vi "Filter_on_template_file_new.vi"(0 "Template File":path, 2 "Extra Channel Values":string[][](array[string]), 3 "Filetype":string, 5 "Channel Names In":string[](array[string]), 9 "Data string":string, 12 "Filename":path) -> (4 "Template File-write":path, 6 "Row numbers":i32[](array[numeric]), 10 "Channel Names Out":string[](array[string]), 14 "Deleted Rows":string[][](array[string]), 15 "Data Out":string[][](array[string]))   [LabVIEW 2021]
panel:
  out "Current Case":string
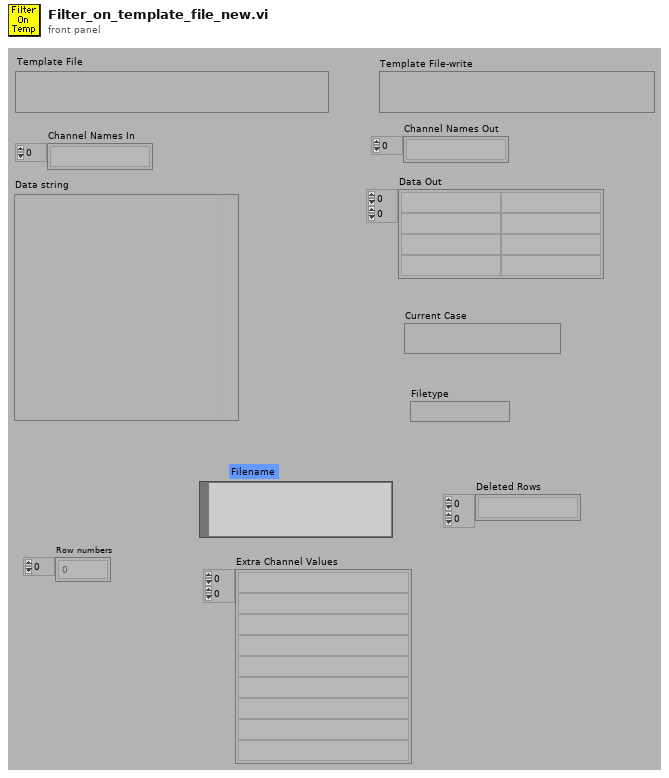
[diagram p1: front panel]
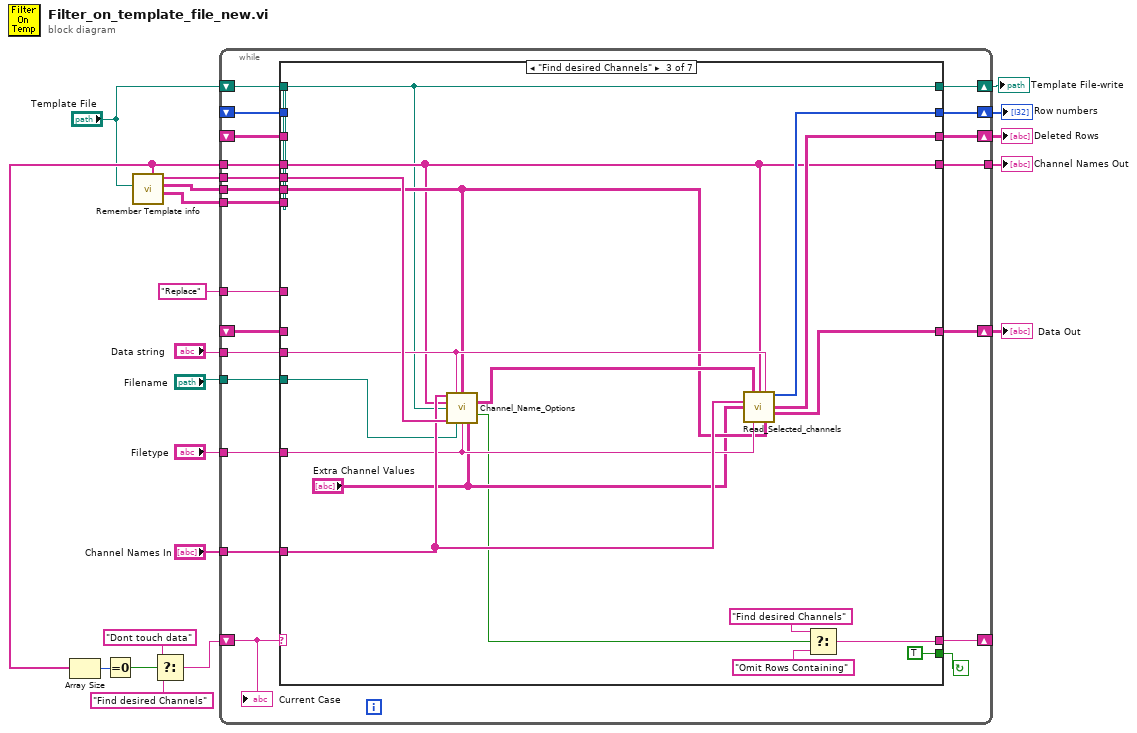
[diagram p0: block diagram]
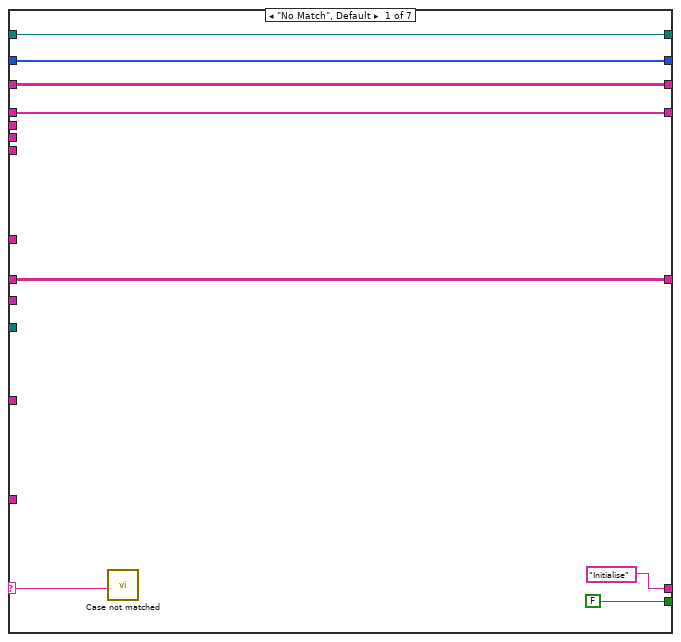
[diagram p2: hidden frame]
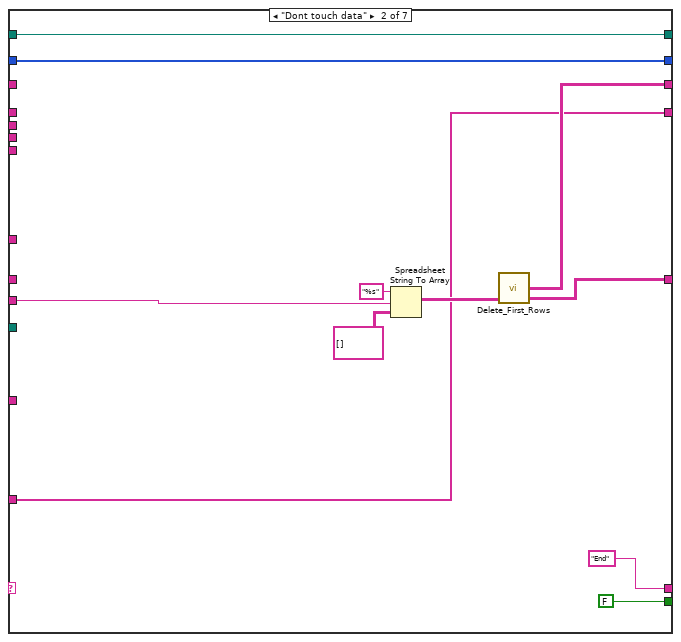
[diagram p3: hidden frame]
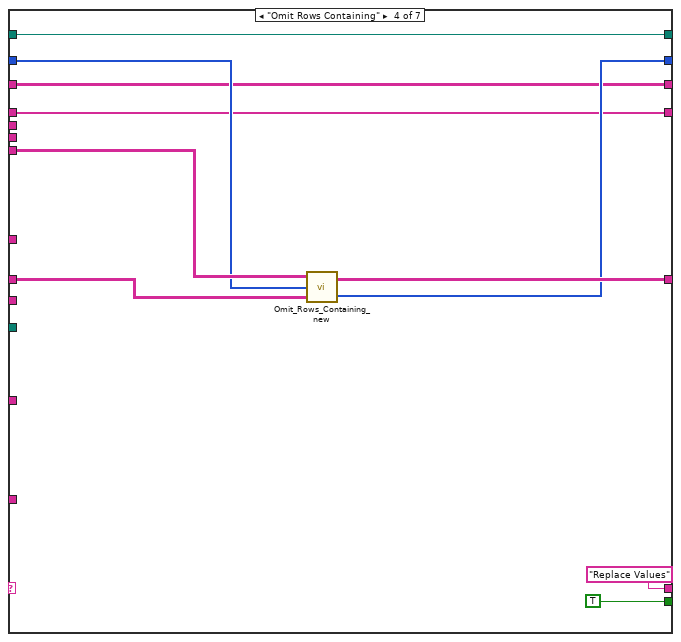
[diagram p4: hidden frame]
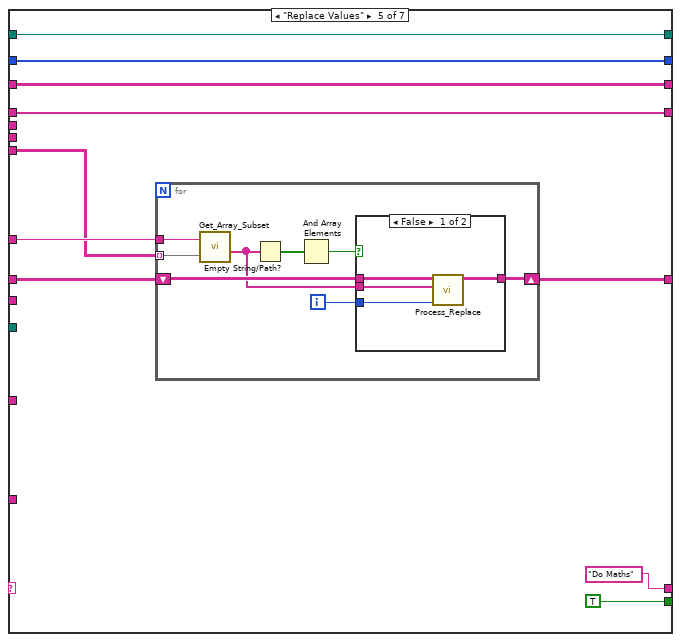
[diagram p5: hidden frame]
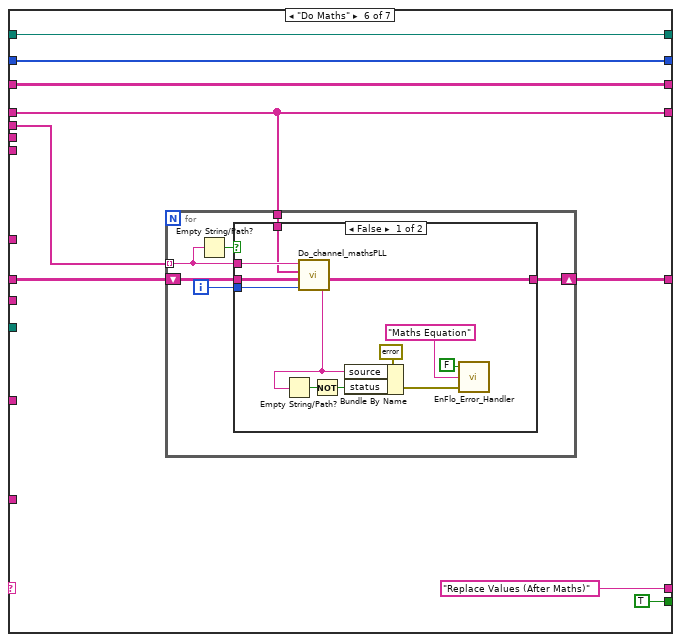
[diagram p7: hidden frame]
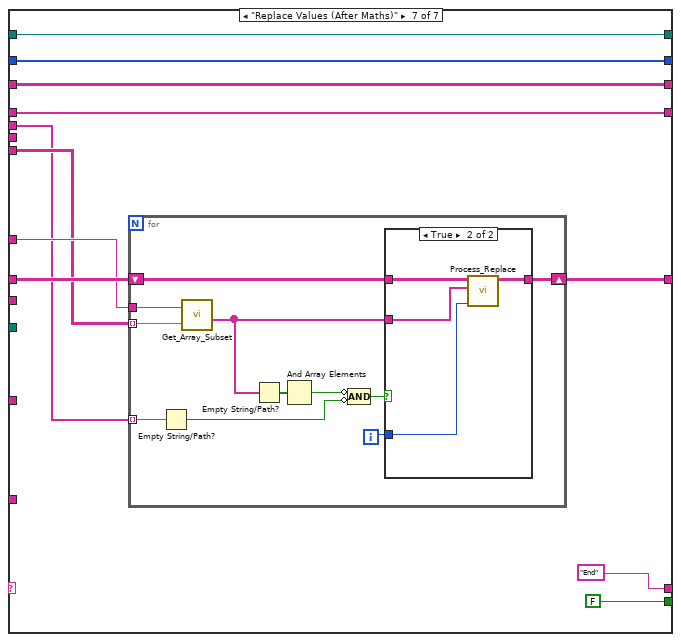
[diagram p9: hidden frame]
diagram:
  n1 = call "Remember Template info.vi"("Template File"="Template File") -> ("2D Template info"=w9:string[][], "Ignore"=w11:string[][], "Maths"=w10:string[], "Template Ch Names Out"=w8:string[])  [unwired: 6 in, 1 out]
  n2 = Array Size(array=w8) -> (size(s)=w7:i32)
  n3 = Equal To 0?(x=w7) -> (x = 0?=w6:bool)
  n4 = Select(t="Dont touch data", s=w6, f="Find desired Channels") -> (s? t:f=w4:string)
  n5 = while {
    tunnel: "Filetype" -> [w21]
    tunnel: "Filename" -> [w32]
    tunnel: "Data string" -> [w33]
    tunnel: "Channel Names In" -> [w34]
    tunnel: "Replace" -> [w35]
    shift-left: _ -> [w36]
    shift-right: [w37] -> w18
    shift-left: "Template File" -> [w38]
    shift-right: [w39] -> w20
    shift-left: w4 -> [w31]
    shift-right: [w40] -> _
    shift-right: [w29] -> w13
    shift-left: _ -> [w30]
    shift-right: [w28] -> w12
    shift-left: _ -> [w27]
    tunnel: w11 -> [w26]
    tunnel: w10 -> [w25]
    tunnel: w9 -> [w24]
    tunnel: w8 -> [w23]
    tunnel: [w22] -> w2
    stop <- w41 continue-if-true
    n6 = case shown="\"Find desired Channels\"" w31 {
      selector: w31 -> [w43 _ _ _ _ _ _]
      tunnel: [FALSE FALSE ("Duplicate rows?") TRUE TRUE TRUE TRUE ("Duplicate rows?") FALSE] -> w41
      tunnel: ["Initialise" "End" w63 "Replace Values" "Do Maths" "Replace Values (After Maths)" "End"] -> w40
      tunnel: [w47 w60 w62 w86 w96 w120 w148] -> w39
      tunnel: w24 -> [_ _ _ w85 w91 _ w143]
      tunnel: w38 -> [w47 w60 w62 w86 w96 w120 w148]
      tunnel: w25 -> [_ _ w77 _ _ w119 w142]
      tunnel: [w46 w53 w74 w83 w95 w115 w147] -> w37
      tunnel: w36 -> [w46 _ _ w84 w94 w116 w146]
      tunnel: w35 -> [_ _ _ _ w92 _ w144]
      tunnel: w34 -> [_ w50 w76 _ _ _ _]
      tunnel: w33 -> [_ w55 w72 _ _ _ _]
      tunnel: w32 -> [_ _ w61 _ _ _ _]
      tunnel: w21 -> [_ _ w73 _ _ _ _]
      tunnel: [w45 w52 w71 w82 w93 w114 w145] -> w29
      tunnel: w30 -> [w45 w52 _ w81 w93 w114 w145]
      tunnel: [w44 w51 w70 w80 w90 w113 w141] -> w28
      tunnel: w27 -> [w44 _ _ w80 w90 w113 w141]
      tunnel: w26 -> [_ _ w69 _ _ _ _]
      tunnel: w23 -> [w42 _ w68 w79 w89 w112 w140]
      tunnel: [w42 w50 w68 w79 w89 w112 w140] -> w22
      frame "No Match", Default {
        n7 = call "Case not matched.vi"("Case Name not Matched"=w43) -> ()
      }
      frame "Dont touch data" {
        n8 = Spreadsheet String To Array(format string="%s", spreadsheet string=w55, array type (2D Dbl)=string[][] [] ("Channel Values")) -> (array=w54:string[][])  [unwired: 1 out]
        n9 = call "Delete_First_Rows.vi"("Data In"=w54) -> ("Deleted Rows"=w51:string[][], "Data Out"=w53:string[][])  [unwired: 1 in, 1 out]
      }
      frame "Find desired Channels" {
        n10 = call "Channel_Name_Options.vi"("All Channel Names"=w76, "Data string"=w72, "Ignore When"=w69, "Template Names"=w68, "Template File"=w62, "Maths In"=w77, "while Reading:"=w61, "Filetype"=w73, "Extra Channel Values"="Extra Channel Values") -> ("Valid Channel Options"=w75:string[][], "Template updated?"=w66:bool)  [unwired: 5 out]
        n11 = call "Read_Selected_channels.vi"("Valid Channel Options"=w75, "Template Names"=w68, "Data string"=w72, "All Channels Present"=w76, "Extra Channels"="Extra Channel Values", "Filetype"=w73, "Ignore When"=w69) -> ("Non-Blank Rows"=w71:i32[], "Deleted Rows"=w70:string[][], "Output Values"=w74:string[][])  [unwired: 5 in, 1 out]
        n12 = Select(t="Find desired Channels", s=w66, f="Omit Rows Containing") -> (s? t:f=w63:string)
      }
      frame "Omit Rows Containing" {
        n13 = call "Omit_Rows_Containing_new.vi"("Data Array In"=w84, "Non-Blank Rows"=w81, "Template Info"=w85) -> ("Row numbers"=w82:i32[], "Data Array Out"=w83:string[][])
      }
      frame "Replace Values" {
        n14 = for {
          shift-right: [w104] -> w95
          shift-left: w94 -> [w105]
          tunnel: w92 -> [w101]
          tunnel: w91 -> [w100] mode=indexing
          i -> [w106]
          n15 = call "Get_Array_Subset.vi"("String Array In"=w100, "Subset Name"=w101) -> ("Array Subset Out"=w99:string[])  [unwired: 4 out]
          n16 = Empty String/Path?(string/path=w99) -> (empty?=w103:bool[])
          n17 = And Array Elements(Boolean array=w103) -> (logical AND=w102:bool)
          n18 = case shown="False" w102 {
            tunnel: w99 -> [w110 _]
            tunnel: w106 -> [w107 _]
            tunnel: w105 -> [w109 w111]
            tunnel: [w108 w111] -> w104
            frame False {
              n19 = call "Process_Replace.vi"("Index"=w107, "Replace array"=w110, "Array In"=w109) -> ("Array Out"=w108:string[][])  [unwired: 1 in, 3 out]
            }
            frame True {
            }
          }
        }
      }
      frame "Do Maths" {
        n20 = for {
          tunnel: w119 -> [w122] mode=indexing
          shift-right: [w124] -> w115
          shift-left: w116 -> [w123]
          tunnel: w112 -> [w121]
          i -> [w125]
          n21 = Empty String/Path?(string/path=w122) -> (empty?=w126:bool)
          n22 = case shown="False" w126 {
            tunnel: w125 -> [w138 _]
            tunnel: [w136 w139] -> w124
            tunnel: w123 -> [w137 w139]
            tunnel: w122 -> [w135 _]
            tunnel: w121 -> [w127 _]
            frame False {
              n23 = call "Do_channel_mathsPLL.vi"("Output Index"=w138, "Channel Values In"=w137, "Channel Names"=w127, "Maths Equation"=w135) -> ("Error String"=w132:string, "Channel Values Out"=w136:string[][])  [unwired: 1 in, 1 out]
              n24 = Empty String/Path?(string/path=w132) -> (empty?=w134:bool)
              n25 = Not(x=w134) -> (.not. x?=w131:bool)
              n26 = Bundle By Name(cluster=errorcluster {"status"=FALSE, "code"=0, "source"=""} ("error in (no error)"), "source"=w132, "status"=w131) -> (w130:errorcluster)
              n27 = call "EnFlo_Error_Handler.vi"("error in (no error)"=w130, "Error Type"="Maths Equation", "Dialog Box (F)"=FALSE ("Dialog Box (T)")) -> ()  [unwired: 3 out]
            }
            frame True {
            }
          }
        }
      }
      frame "Replace Values (After Maths)" {
        n28 = for {
          shift-right: [w159] -> w147
          shift-left: w146 -> [w160]
          tunnel: w144 -> [w157]
          tunnel: w143 -> [w156] mode=indexing
          tunnel: w142 -> [w152] mode=indexing
          i -> [w161]
          n29 = Empty String/Path?(string/path=w152) -> (empty?=w151:bool)
          n30 = call "Get_Array_Subset.vi"("String Array In"=w156, "Subset Name"=w157) -> ("Array Subset Out"=w155:string[])  [unwired: 4 out]
          n31 = Empty String/Path?(string/path=w155) -> (empty?=w158:bool[])
          n32 = And Array Elements(Boolean array=w158) -> (logical AND=w154:bool)
          n33 = Compound Arithmetic op=AND(invert w154, invert w151) -> (w153:bool)
          n34 = case shown="True" w153 {
            tunnel: w155 -> [_ w166]
            tunnel: w161 -> [_ w163]
            tunnel: w160 -> [w162 w165]
            tunnel: [w162 w164] -> w159
            frame False {
            }
            frame True {
              n35 = call "Process_Replace.vi"("Index"=w163, "Replace array"=w166, "Array In"=w165) -> ("Array Out"=w164:string[][])  [unwired: 1 in, 3 out]
            }
          }
        }
      }
    }
    "Current Case" <- w31
  }
  "Channel Names Out" <- w2
  "Data Out" <- w18
  "Template File-write" <- w20
  "Row numbers" <- w13
  "Deleted Rows" <- w12
